vi "read_position.vi"(8 "error in (no error)":errorcluster, 11 "VISA Refnum in":refnum<visa-resource-name>) -> (0 "error out":errorcluster, 1 "Moving":bool, 2 "Position":i32, 3 "VISA Refnum out":refnum<visa-resource-name>)   [LabVIEW 2015]
panel:
  out "Moving State":i32
  out "read buffer":string
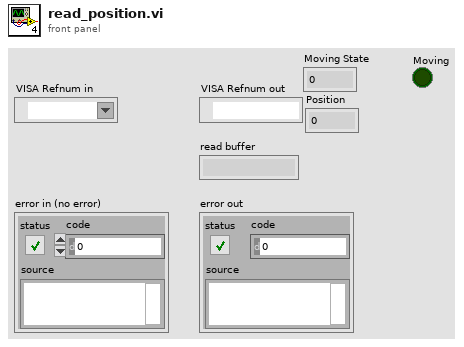
[diagram p1: front panel]
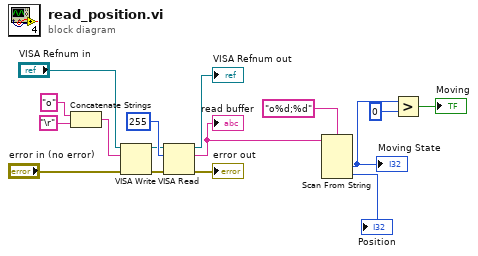
[diagram p0: block diagram]
diagram:
  n1 = Concatenate Strings("o" ("write buffer"), "\r") -> (w1:string)
  n2 = VISA Write(VISA resource name="VISA Refnum in", write buffer=w1, error in (no error)="error in (no error)") -> (VISA resource name out=w9:refnum<visa-resource-name>, error out=w15:errorcluster)  [unwired: 1 out]
  n3 = VISA Read(VISA resource name=w9, byte count=u32 255, error in (no error)=w15) -> (VISA resource name out=→"VISA Refnum out":refnum<visa-resource-name>, read buffer=w8:string, error out=→"error out":errorcluster)  [unwired: 1 out]
  "read buffer" <- w8
  n4 = Scan From String(format string="o%d;%d", input string=w8) -> (output 1=w5:i32, output 2=→"Position":i32)  [unwired: 4 in, 3 out]
  "Moving State" <- w5
  n5 = Greater?(x=w5, y=0) -> (0:→"Moving":bool)
